vi "Destroy.vi"(8 "error in":errorcluster, 11 "Buffer Lossless DBL in":refnum<class "Buffer Lossless DBL.lvclass">) -> (0 "error out":errorcluster, 3 "Buffer Lossless DBL out":refnum<class "Buffer Lossless DBL.lvclass">)   [LabVIEW 2024, in "Buffer Lossless DBL.lvclass"]
uses:
  Buffer Lossless DBL.lvclass
  Buffer Lossless DBL.lvclass/Buffer Lossless DBL.ctl
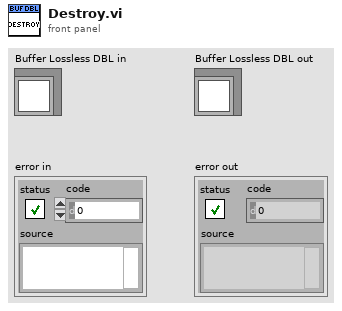
[diagram p1: front panel]
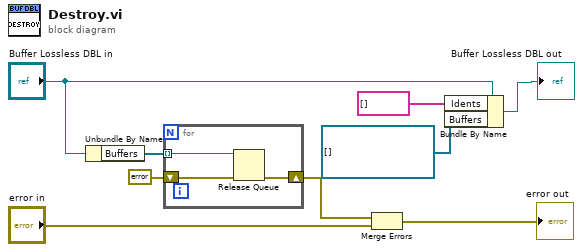
[diagram p0: block diagram]
diagram:
  n1 = Unbundle By Name("Buffer Lossless DBL in") -> ("Buffers"=w9:refnum<queue>[])
  n2 = for {
    tunnel: w9 -> [w12] mode=indexing
    shift-right: [w11] -> w7
    shift-left: errorcluster {"status"=FALSE, "code"=0, "source"=""} ("error out") -> [w10]
    n3 = Release Queue(queue=w12, error in (no error)=w10) -> (error out=w11:errorcluster)  [unwired: 1 in, 2 out]
  }
  n4 = Merge Errors(w7, "error in") -> (→"error out":errorcluster)
  n5 = Bundle By Name(cluster="Buffer Lossless DBL in", "Idents"=string[] [], "Buffers"=refnum<queue>[] []) -> (→"Buffer Lossless DBL out":refnum<class "Buffer Lossless DBL.lvclass">)
